vi "Toggle.vi"(7 "Control":bool=TRUE, 10 "Input":bool) -> (2 "Output":bool)   [LabVIEW 2017]
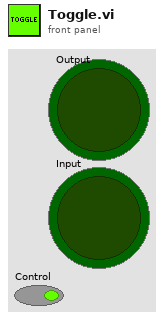
[diagram p1: front panel]
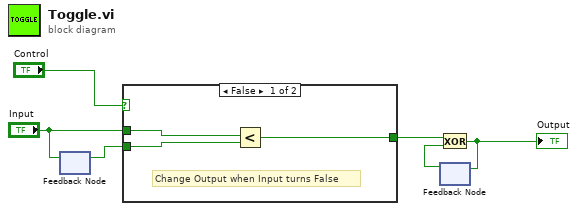
[diagram p0: block diagram]
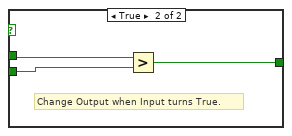
[diagram p2: hidden frame]
diagram:
  n1 = feedback #1() -> (w4:bool)  [unwired: 1 in]
  n2 = feedback-in #1("Input") -> ()
  n3 = case shown="False" "Control" {
    tunnel: [w9 w12] -> w5
    tunnel: w4 -> [w8 w10]
    tunnel: "Input" -> [w7 w11]
    frame False {
      # "Change Output when Input turns False"
      n4 = Less?(x=w7, y=w8) -> (x < y?=w9:bool)
    }
    frame True {
      # "Change Output when Input turns True."
      n5 = Greater?(x=w11, y=w10) -> (0:w12:bool)
    }
  }
  n6 = feedback #2() -> (w6:bool)  [unwired: 1 in]
  n7 = Exclusive Or(1:w6, 2:w5) -> (0:w1:bool)
  "Output" <- w1
  n8 = feedback-in #2(w1) -> ()
